vi "Log DAC Cmd.vi"(8 "error in":errorcluster, 10 "DAC Process Command in":refnum<class "Generic DAC Process Command.lvclass">, 11 "DAC Process Data in":T1) -> (0 "error out":errorcluster, 3 "DAC Process Data out":T1)   [LabVIEW 2019, in "DAC Process.lvlib" / "Generic DAC Process Command.lvclass"]
uses:
  Generic DAC Process Command.lvclass
  DAC Process Data.ctl
  Generic Test Stand/Generic Test Stand.lvclass
  TS Framework/ExeLogging/DAC Logger/DAC Logger.lvclass
  DAC State.ctl
  Generic DAC Process Command.lvclass/Generic DAC Process Command.ctl
  DAC Process.lvlib
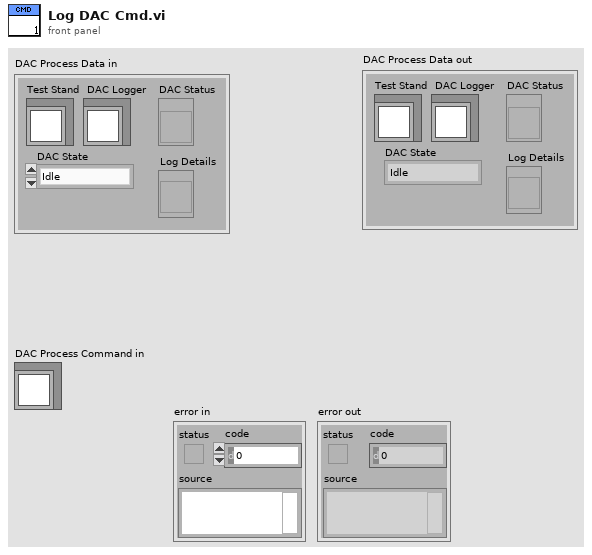
[diagram p1: front panel]
types:
  T1 = typedef "DAC Process.lvlib/DAC Process Data.ctl" = cluster{"Test Stand":refnum<class "Generic Test Stand.lvclass">, " DAC Logger":refnum<class "DAC Logger.lvclass">, "DAC State":T2, "DAC Status":refnum<vi>, "Log Details":refnum<vi>}
  T2 = typedef "DAC Process.lvlib/DAC State.ctl" = enum16{"Idle", "Acquiring"}
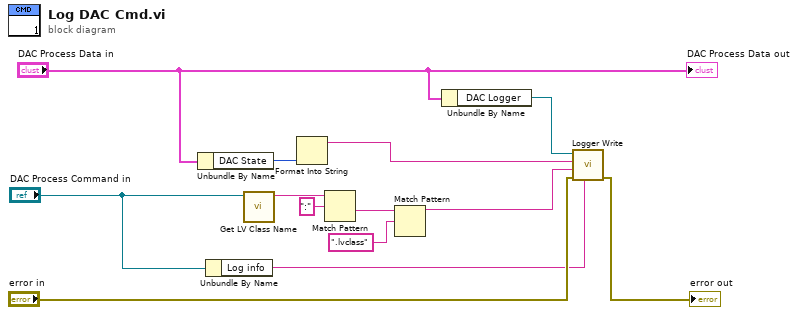
[diagram p0: block diagram]
diagram:
  n1 = Unbundle By Name("DAC Process Data in") -> ("DAC State"=w7:T2)
  n2 = Unbundle By Name("DAC Process Command in") -> ("Log info"=w8:string)
  n3 = call <vilib>:"Get LV Class Name.vi"("object"="DAC Process Command in") -> ("class name"=w10:string)  [unwired: 9 in, 1 out]
  n4 = Format Into String(w7) -> (resulting string=w6:string)  [unwired: 3 in, 1 out]
  n5 = Match Pattern(string=w10, regular expression=":") -> (after substring=w5:string)  [unwired: 1 in, 3 out]
  n6 = Match Pattern(string=w5, regular expression=".lvclass") -> (before substring=w3:string)  [unwired: 1 in, 3 out]
  n7 = Unbundle By Name("DAC Process Data in") -> ("DAC Logger"=w11:refnum<class "DAC Logger.lvclass">)
  n8 = call-dynamic "Logger Write.vi"("Extra"=w8, "error in (no error)"="error in", "Command"=w3, "State"=w6, "Logger in"=w11) -> ("error out"=→"error out":errorcluster)  [unwired: 6 in]
  "DAC Process Data out" <- "DAC Process Data in"
